vi "Load_from_Project.vi"(8 "error in (no error)":errorcluster, 9 "index in":string, 10 "buildObject":T1, 11 "IB_Source_Container in":refnum<class "IB_Source_Container.lvclass">) -> (0 "error out":errorcluster, 1 "index out":string, 2 "buildObject out":T1, 3 "IB_Source_Container out":refnum<class "IB_Source_Container.lvclass">)   [LabVIEW 2020, in "IB_Source_Container.lvclass"]
uses:
  <vilib>/AppBuilder/IB_Classes/Source/Container/IB_Source_Container.lvclass
  <vilib>/AppBuilder/IB_Classes/Source/Container/IB_Source_Container.lvclass/IB_Source_Container.ctl
  <vilib>/AppBuilder/IB_Classes/Source/IB_Source.lvclass
  <vilib>/AppBuilder/IB_Classes/Source/File/CtrFile/IB_CtrFile.lvclass
  <resource>/Framework/Providers/API/ItemRef.ctl
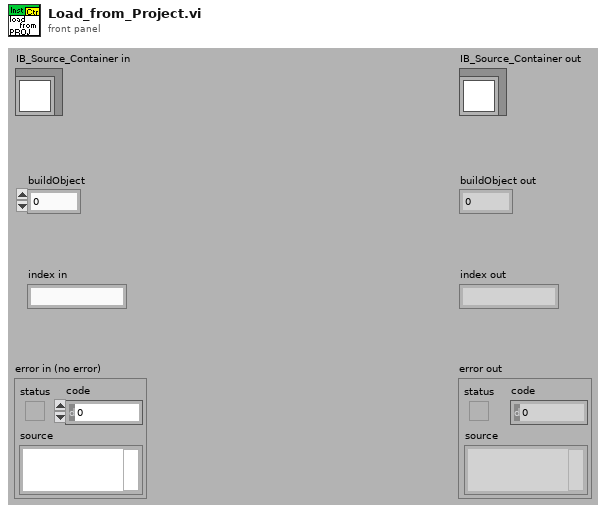
[diagram p1: front panel]
types:
  T1 = typedef "ItemRef.ctl" = u64
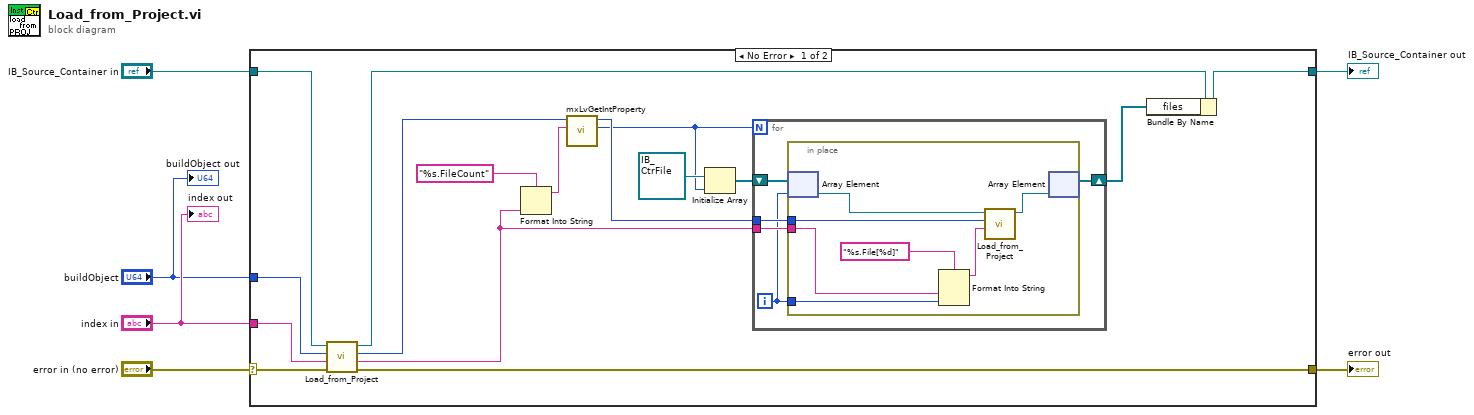
[diagram p0: block diagram]
diagram:
  n1 = case shown="No Error" "error in (no error)" {
    selector: "error in (no error)" -> [w18 w36]
    tunnel: [w22 w36] -> w4
    tunnel: [w9 w35] -> w3
    tunnel: "index in" -> [w21 _]
    tunnel: "buildObject" -> [w20 _]
    tunnel: "IB_Source_Container in" -> [w19 w35]
    frame No Error {
      n2 = call-parent "Load_from_Project.vi"("error in (no error)"=w18, "index in"=w21, "buildObject"=w20, "IB_Source in"=w19) -> ("error out"=w22:errorcluster, "index out"=w8:string, "buildObject out"=w7:T1, "IB_Source out"=w10:refnum<class "IB_Source_Container.lvclass">)  [unwired: 4 in]
      n3 = Format Into String(format string="%s.FileCount", w8) -> (resulting string=w16:string)  [unwired: 2 in, 1 out]
      n4 = call <resource>:"mxLvGetIntProperty.vi"("Tag"=w16, "Item"=w7) -> ("Value"=w12:i32, "Item"=w15:T1)  [unwired: 1 in, 7 out]
      n5 = Initialize Array(refnum<class "IB_CtrFile.lvclass"> refnum ("IB_CtrFile.lvclass"), w12) -> (w13:refnum<class "IB_CtrFile.lvclass">[])
      n6 = for {
        N: w12 -> [_]
        tunnel: w8 -> [w27]
        tunnel: w15 -> [w26]
        shift-right: [w24] -> w11
        shift-left: w13 -> [w25]
        i -> [w23]
        n7 = in-place {
          in-place-border: w27 -> [w29]
          in-place-border: w26 -> [w34]
          in-place-border: w23 -> [w30]
          n8 = in-place-array #1(w25, w23) -> (w33:refnum<class "IB_CtrFile.lvclass">)
          n9 = Format Into String(format string="%s.File[%d]", w29, w30) -> (resulting string=w28:string)  [unwired: 2 in, 1 out]
          n10 = call-dynamic "Load_from_Project.vi"("index"=w28, "buildObject"=w34, "IB_Source_File in"=w33) -> ("IB_Source_File out"=w32:refnum<class "IB_CtrFile.lvclass">)  [unwired: 5 in, 3 out]
          n11 = in-place-array #1(w32) -> (w24:refnum<class "IB_CtrFile.lvclass">[])  [unwired: 1 out]
        }
      }
      n12 = Bundle By Name(cluster=w10, "files"=w11) -> (w9:refnum<class "IB_Source_Container.lvclass">)
    }
    frame Error {
    }
  }
  "error out" <- w4
  "IB_Source_Container out" <- w3
  "buildObject out" <- "buildObject"
  "index out" <- "index in"
